vi "34970 Error Query (Multiple)+++.vi"(0 "VISA resource name":refnum<visa-resource-name>, 11 "error in (no error)":errorcluster) -> (4 "VISA resource name out":refnum<visa-resource-name>, 8 "Error":i32[](array[numeric]), 10 "Error Message":string, 15 "error out":errorcluster)   [LabVIEW 2020]
doc: "This VI reads the error queue from the instrument. It expects to see errors in SCPI format (#,\"error message\"). It continues to read from the error queue until it reads a 0, \"No error\". If the instrument does not support an error query, a warning is returned."
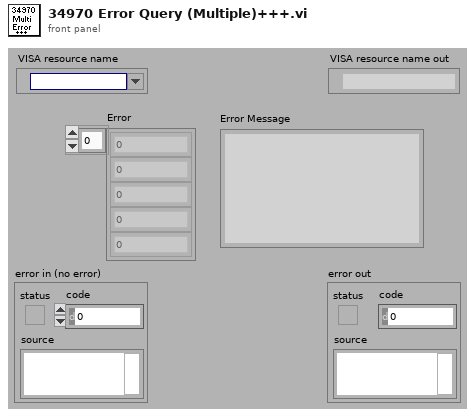
[diagram p1: front panel]
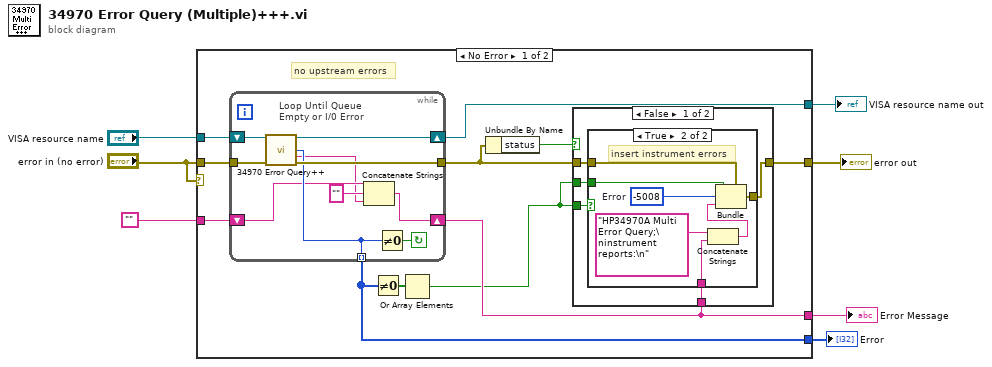
[diagram p0: block diagram]
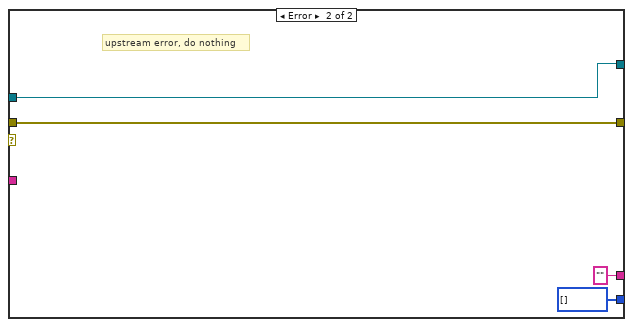
[diagram p4: hidden frame]
diagram:
  n1 = case shown="No Error" "error in (no error)" {
    tunnel: "" ("Empty String Constant") -> [w18 _]
    tunnel: [w17 ""] -> w7
    tunnel: [w14 w46] -> w6
    tunnel: [w13 w45] -> w5
    tunnel: "error in (no error)" -> [w12 w45]
    tunnel: "VISA resource name" -> [w11 w46]
    tunnel: [w8 i32[] []] -> w1
    frame No Error {
      # "no upstream errors"
      n2 = while {
        shift-right: [w22] -> w17
        shift-left: w18 -> [w21]
        shift-right: [w28] -> w14
        shift-left: w11 -> [w26]
        tunnel: [w25] -> w16
        tunnel: [w23] -> w8 mode=indexing
        tunnel: w12 -> [w24]
        stop <- w27 continue-if-true
        # "Loop Until Queue Empty or I/0 Error"
        n3 = call "34970 Error Query++.vi"("VISA session"=w26, "error in (no error)"=w24) -> ("dup VISA session"=w28:refnum<visa-resource-name>, "Error"=w23:i32, "Error Message"=w19:string, "error out"=w25:errorcluster)  [unwired: 10 in]
        n4 = Concatenate Strings(w21, "" ("string"), w19) -> (w22:string)
        n5 = Not Equal To 0?(x=w23) -> (x != 0?=w27:bool)
      }
      n6 = Not Equal To 0?(x=w8) -> (x != 0?=w10:bool[])
      n7 = Or Array Elements(Boolean array=w10) -> (logical OR=w9:bool)
      n8 = Unbundle By Name(w16) -> ("status"=w15:bool)
      n9 = case shown="False" w15 {
        tunnel: w16 -> [w33 w42]
        tunnel: [w32 w42] -> w13
        tunnel: w17 -> [w29 _]
        tunnel: w9 -> [w31 _]
        tunnel: w9 -> [w30 _]
        frame False {
          n10 = case shown="True" w30 {
            tunnel: w33 -> [w34 w40]
            tunnel: [w34 w39] -> w32
            tunnel: w31 -> [_ w36]
            tunnel: w29 -> [_ w35]
            frame False {
              # "no instrument errors"
            }
            frame True {
              w41 = -5008  # Error
              # "insert instrument errors"
              n11 = Concatenate Strings("HP34970A Multi Error Query;\ninstrument reports:\n", w35) -> (w38:string)
              n12 = Bundle(cluster=w40, "status"=w36, "code"=w41, "source"=w38) -> (w39:errorcluster)
            }
          }
        }
        frame True {
          # "upstream error or comm\nproblem w/query"
        }
      }
    }
    frame Error {
      # "upstream error, do nothing"
    }
  }
  "Error Message" <- w7
  "error out" <- w5
  "VISA resource name out" <- w6
  "Error" <- w1
